vi "SeqMgr.Result, Update Result State based on Error Event.vi"(10 "error in":errorcluster, 11 "Result Info":T1={"State"=enum."PASS", "Code"=0, "Description"=""}) -> (3 "Result Info Out":T1={"State"=enum."PASS", "Code"=0, "Description"=""})   [LabVIEW 2024, in "EQMF.lvlib" / "SeqMgr.lvlib"]
uses:
  SeqMgr.lvlib
  SeqMgr.Result Info.ctl
  SeqMgr.Result State Enum.ctl
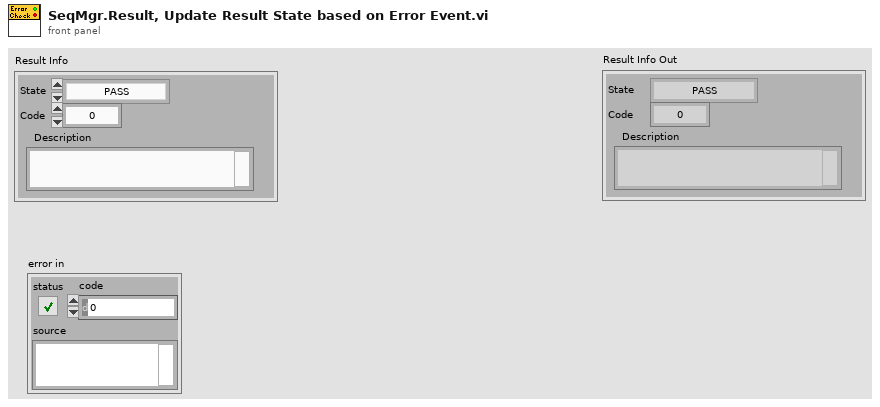
[diagram p1: front panel]
types:
  T1 = typedef "EQMF.lvlib/SeqMgr.lvlib/SeqMgr.Result Info.ctl" = cluster{"State":T2, "Code":i32, "Description":string}
  T2 = typedef "EQMF.lvlib/SeqMgr.lvlib/SeqMgr.Result State Enum.ctl" = enum16{"None", "Passing", "Failing", "PASS", "FAIL", "ABORT", "ERROR"}
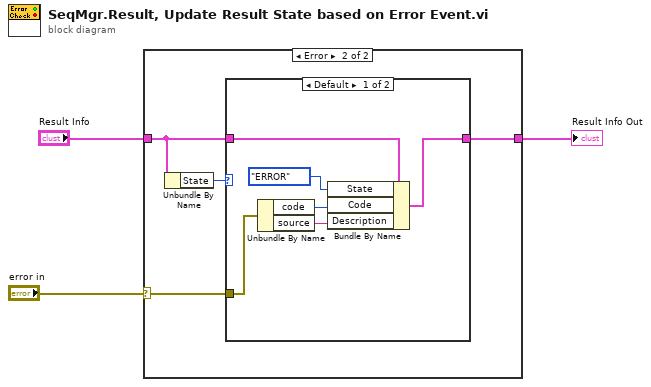
[diagram p0: block diagram]
diagram:
  n1 = case shown="Error" "error in" {
    selector: "error in" -> [_ w5]
    tunnel: "Result Info" -> [w4 w7]
    tunnel: [w4 w6] -> w1
    frame No Error {
    }
    frame Error {
      n2 = Unbundle By Name(w7) -> ("State"=w8:T2)
      n3 = case shown="Default" w8 {
        tunnel: w7 -> [w14 w15]
        tunnel: [w12 w15] -> w6
        tunnel: w5 -> [w11 _]
        frame Default {
          n4 = Unbundle By Name(w11) -> ("code"=w10:i32, "source"=w9:string)
          n5 = Bundle By Name(cluster=w14, "State"=SeqMgr.Result_State_Enum."ERROR", "Code"=w10, "Description"=w9) -> (w12:T1)
        }
        frame "ERROR" {
          # "No Change"
        }
      }
    }
  }
  "Result Info Out" <- w1
